vi "Send Set UI VI Reference.vi"(7 "Priority":T1=enum."Normal" caption="Message Priority (Normal)", 8 "error in (no error)":errorcluster, 10 "UI VI Reference (caller)":refnum<vi>, 11 "Message Enqueuer in":refnum<class "Message Enqueuer.lvclass">) -> (0 "error out":errorcluster, 3 "Message Enqueuer out":refnum<class "Message Enqueuer.lvclass">)   [LabVIEW 2014, in "Flex UI (Parent Actor).lvlib" / "Set UI VI Reference Msg.lvclass"]
doc: "Sends the <b>Set UI VI Reference Msg.lvclass</b> message.\n\nThis message will call <b>Set UI VI Reference.vi</b> on the <b>Flex UI (Parent Actor).lvlib:Flex UI (Actor).lvclass</b> actor.\n\n<b>Set UI VI Reference.vi Description</b>\nWrapper around the Set UI VI Reference method within the Flex UI class. This sets the UI VI Reference that resides in the private data of the Flex UI class."
uses:
  Set UI VI Reference Msg.lvclass
  <vilib>/ActorFramework/Message Enqueuer/Message Enqueuer.lvclass
  <vilib>/ActorFramework/Message Enqueuer/Message Priority.ctl
  Set UI VI Reference Msg.lvclass/Set UI VI Reference Msg.ctl
  <vilib>/ActorFramework/Message Enqueuer/Message Enqueuer.lvclass/Message Enqueuer.ctl
  <vilib>/ActorFramework/Message Priority Queue/Priority Enqueue.vi
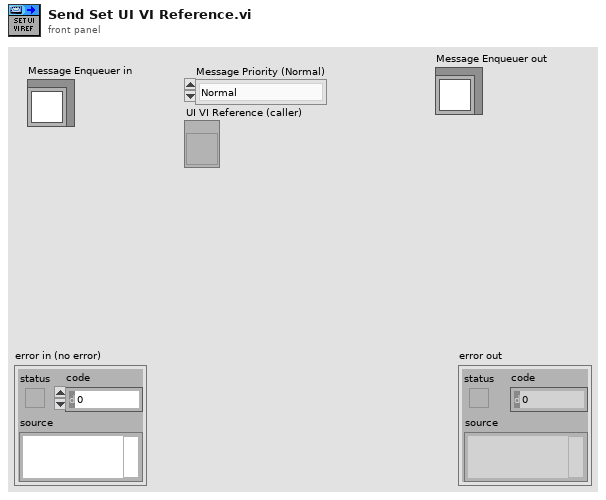
[diagram p1: front panel]
types:
  T1 = typedef "Actor Framework.lvlib/Message Enqueuer.lvclass/Message Priority.ctl" = enum16{"Low", "Normal", "High"}
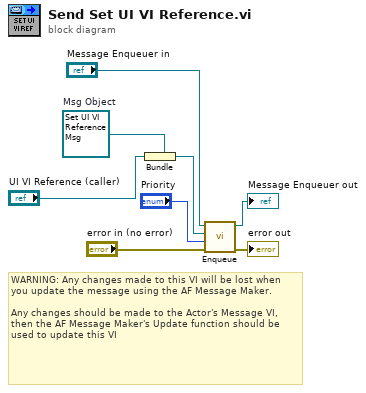
[diagram p0: block diagram]
diagram:
  w7 = refnum<class "Set UI VI Reference Msg.lvclass"> refnum  # Msg Object
  # "WARNING: Any changes made to this VI will be lost when you update the message using the AF Message Maker.\n\nAny changes should be made to the Actor's Message VI, then the AF Message Maker's Update function should be used to update this VI"
  n1 = Bundle(cluster=w7, "UI VI Reference (caller)") -> (w2:refnum<class "Set UI VI Reference Msg.lvclass">)
  n2 = call <vilib>:"Enqueue.vi"("error in (no error)"="error in (no error)", "Message Priority (Normal)"="Priority", "Message"=w2, "Message Enqueuer in"="Message Enqueuer in") -> ("error out"=→"error out":errorcluster, "Message Enqueuer out"=→"Message Enqueuer out":refnum<class "Message Enqueuer.lvclass">)  [unwired: 6 in]
